vi "Obtain Drive Lock.vi"(8 "error in":errorcluster, 11 "Queue in":refnum<queue>) -> (0 "error out":errorcluster, 1 "notifier out":refnum<notifier>, 2 "Lock":string, 3 "queue out":refnum<queue>)   [LabVIEW 2016, in "Drive System.lvlib"]
uses:
  Drive System.lvlib
  DriveCmd.ctl
  DriveCmdList.ctl
  Varient Cmd Types/Lock Command.ctl
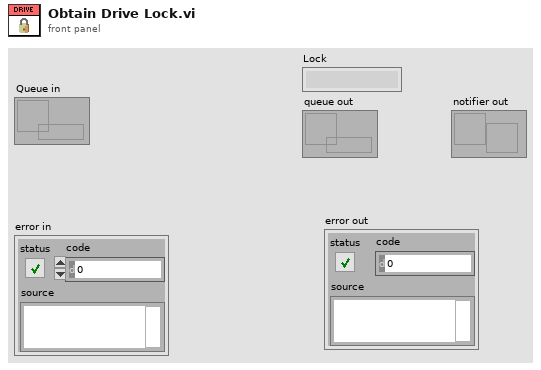
[diagram p1: front panel]
types:
  T1 = typedef "Drive System.lvlib/Lock Command.ctl" = cluster{"notifier out":refnum<notifier>}
  T2 = typedef "Drive System.lvlib/DriveCmd.ctl" = cluster{"cmd":T3, "data":variant, "Force? (F)":bool, "Lock":string}
  T3 = typedef "Drive System.lvlib/DriveCmdList.ctl" = enum16{"Idle", "Cleanup", "Drive For Time", "Follow Path", "Drive Tank", "Drive Arcade", "Unlock", "Lock"}
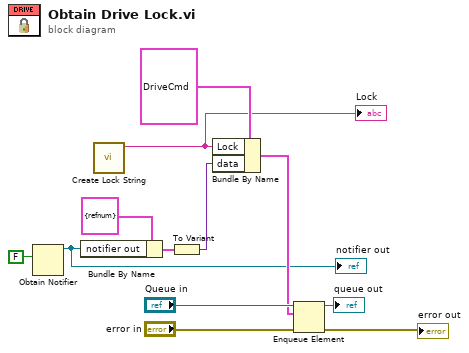
[diagram p0: block diagram]
diagram:
  n1 = Obtain Notifier(notification data type=FALSE) -> (notifier out=w4:refnum<notifier>)  [unwired: 3 in, 2 out]
  "notifier out" <- w4
  n2 = Bundle By Name(cluster=T1 {"notifier out"=refnum} ("Cluster"), "notifier out"=w4) -> (w2:T1)
  n3 = call "Create Lock String.vi"() -> ("String"=w7:string)  [unwired: 11 in]
  "Lock" <- w7
  n4 = To Variant(anything=w2) -> (Variant=w1:variant)
  n5 = Bundle By Name(cluster=T2 {"cmd"=enum."Lock", "data"=variant, "Force? (F)"=FALSE, "Lock"=""} ("element"), "Lock"=w7, "data"=w1) -> (w8:T2)
  n6 = Enqueue Element(queue="Queue in", element=w8, error in (no error)="error in") -> (queue out=→"queue out":refnum<queue>, error out=→"error out":errorcluster)  [unwired: 1 in, 1 out]
